vi "对中 二分法.vi"(8 "error in (no error)":errorcluster caption="错误输入（无错误）", 11 "信号数据":dbl[][](array[numeric])) -> (0 "error out":errorcluster caption="错误输出")   [LabVIEW 2015, in "Logging.lvlib"]
uses:
  Logging.lvlib
  <vilib>/Analysis/NI_AALBase.lvlib
  <vilib>/Analysis/baseanly.llb/Mean (DBL).vi
panel:
  out "转动？":bool
  out "偏差角度":dbl format="%0.2f"
  out "偏差扭矩":dbl format="%0.2f"
  in  "取消按钮":bool
  in  "确定按钮":bool
  # "对称测量结果"
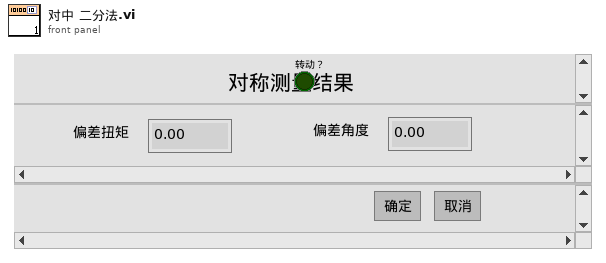
[diagram p1: front panel]
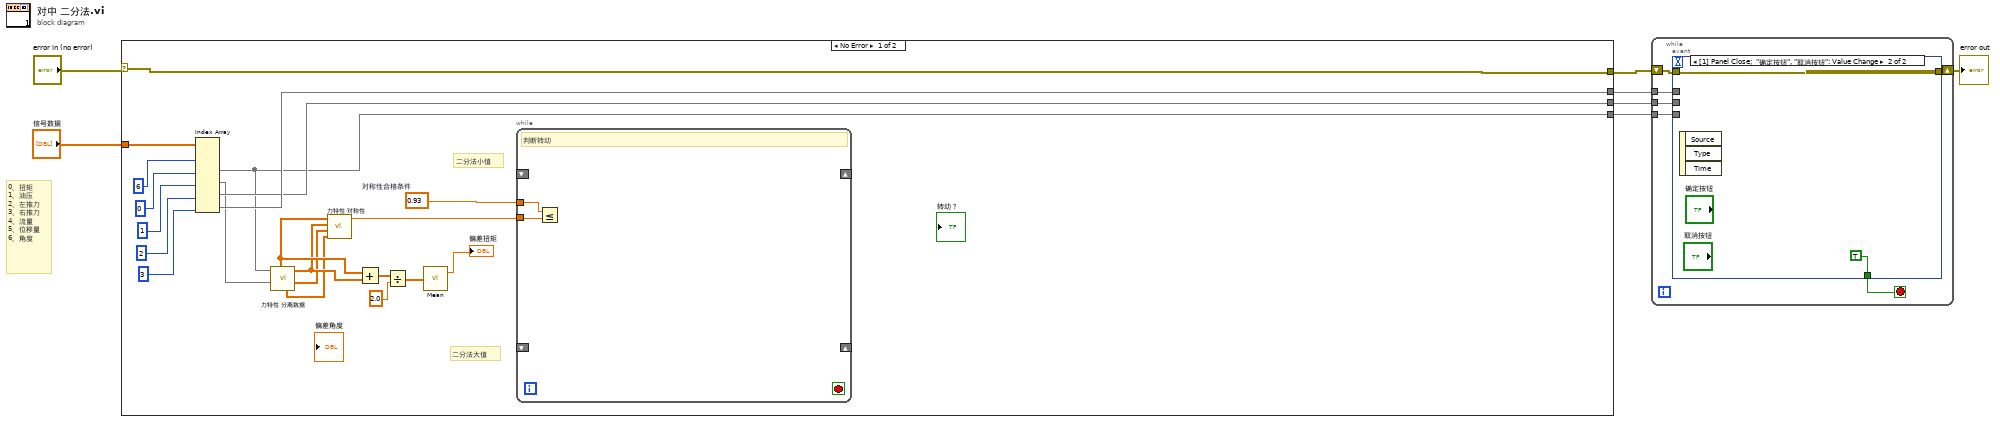
[diagram p0: block diagram]
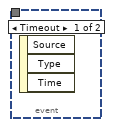
[diagram p2: hidden frame]
diagram:
  # "0、扭矩\n1、油压\n2、左推力\n3、右推力\n4、流量\n5、位移量\n6、角度"
  n1 = case shown="No Error" "error in (no error)" {
    selector: "error in (no error)" -> [w27 w31]
    tunnel: "信号数据" -> [w28 _]
    tunnel: [w27 w31] -> w5
    tunnel: [w26 _] -> w3
    tunnel: [w25 _] -> w2
    tunnel: [w19 _] -> w1
    frame No Error {
      w8 = 0.93  # 对称性合格条件
      # "二分法大值"
      # "二分法小值"
      n2 = Index Array(array=w28, index (col) #1=6 ("禁用的索引 (列)"), index (col) #2=0 ("索引 (行)"), index (col) #3=1 ("索引 (行)"), index (col) #4=2 ("索引 (行)"), index (col) #5=3 ("索引 (行)")) -> (element #2=w19:dbl[], element #3=w18:dbl[], element #4=w25:dbl[], element #5=w26:dbl[])  [unwired: 5 in, 1 out]
      n3 = call "力特性 分离数据.vi"("油压"=w18, "扭矩"=w19) -> ("油压正转去"=w11:dbl[], "扭矩反转去"=w12:dbl[], "油压反转去"=w10:dbl[], "扭矩正转去"=w13:dbl[])  [unwired: 2 in, 4 out]
      n4 = call "力特性 对称性.vi"("油压B"=w10, "油压A"=w11, "扭矩B"=w12, "扭矩A"=w13) -> ("对称性"=w9:dbl)  [unwired: 7 in]
      n5 = Add(x=w13, y=w12) -> (x+y=w17:dbl[])
      n6 = Divide(x=w17, y=2.0) -> (x/y=w15:dbl[])
      n7 = call-poly <vilib>:"Mean.vi"("X"=w15) -> ("mean"=→"偏差扭矩":dbl)  [unwired: 1 out]
      n8 = while {
        shift-right: _ -> [_]
        shift-left: _ -> [_]
        shift-right: _ -> [_]
        shift-left: _ -> [_]
        tunnel: w9 -> [w30]
        tunnel: w8 -> [w29]
        stop <- _ stop-if-true
        # "判断转动"
        n9 = Less Or Equal?(x=w29, y=w30) -> ()  [unwired: 1 out]
      }
    }
    frame Error {
    }
  }
  n10 = while {
    shift-right: [w36] -> w4
    shift-left: w5 -> [w37]
    tunnel: w3 -> [w33]
    tunnel: w2 -> [w32]
    tunnel: w1 -> [w34]
    stop <- w35 stop-if-true
    n11 = event shown="[1] Panel Close;  \"确定按钮\", \"取消按钮\": Value Change" {
      selector: _ -> [_ _]
      dyn-events: _ -> [_ _]
      timeout: _ -> [_ _]
      tunnel: w37 -> [_ w39]
      tunnel: [_ w39] -> w36
      tunnel: [_ TRUE] -> w35
      tunnel: w34 -> [_ _]
      tunnel: w33 -> [_ _]
      tunnel: w32 -> [_ _]
      event Timeout {
        n12 = event-data() -> ()  [unwired: 1 in, 3 out]
      }
      event Panel Close; "确定按钮", "取消按钮": Value Change {
        n13 = event-data() -> ()  [unwired: 1 in, 3 out]
      }
    }
  }
  "error out" <- w4
